vi "Find Labjack.vi"() -> (3 "Instrument Driver":refnum<class "Instrument Driver.lvclass">)   [LabVIEW 2021]
uses:
  LabJack Driver.lvclass
  C:/Git/NHMFL_Core/Libraries/Instruments/Simple VISA Reader/Simple VISA Reader Driver.lvclass
  C:/Git/NHMFL_Core/Libraries/Instruments/VISA Instrument/VISA Instrument.lvclass
  C:/Git/NHMFL_Core/Libraries/Instruments/Instrument Driver/Instrument Driver.lvclass
  C:/Git/NHMFL_Core/Libraries/Instruments/LabJack/LabJack Driver.lvclass
  Instrument Driver/Instrument Driver.lvclass
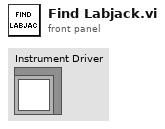
[diagram p1: front panel]
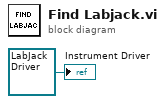
[diagram p0: block diagram]
diagram:
  "Instrument Driver" <- refnum<class "LabJack Driver.lvclass"> refnum ("LabJack Driver.lvclass")
